vi "AlarmText.vi"(11 "Input":i32) -> (3 "Output":string)   [LabVIEW 2014]
doc: "Create text to add a our .txt files"
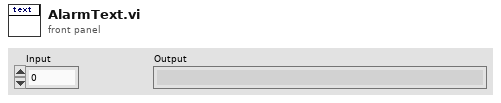
[diagram p1: front panel]
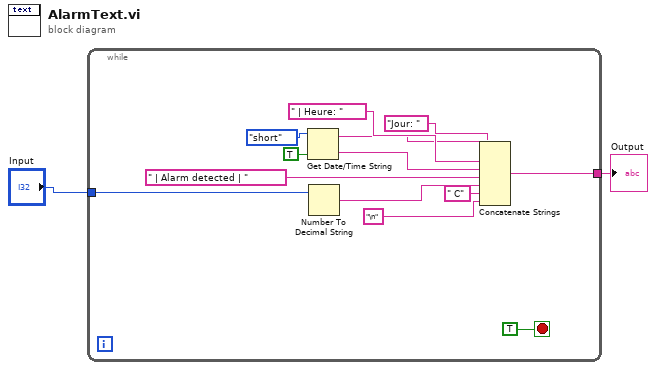
[diagram p0: block diagram]
diagram:
  n1 = while {
    tunnel: "Input" -> [w4]
    tunnel: [w3] -> w1
    stop <- TRUE stop-if-true
    n2 = Get Date/Time String(date format (0)=enum16{"short", "long", "abbreviated"}."short", want seconds? (F)=TRUE) -> (date string=w12:string, time string=w14:string)  [unwired: 1 in]
    n3 = Number To Decimal String(number=w4) -> (decimal integer string=w9:string)  [unwired: 1 in]
    n4 = Concatenate Strings("Jour: " ("string"), w12, " | Heure: " ("string"), w14, " | Alarm detected | " ("string"), w9, " C" ("string"), "\n" ("string")) -> (w3:string)
  }
  "Output" <- w1
